vi "Action2Target.vi"() -> ()   [LabVIEW 2017]
panel:
  in  "Current":dbl
  in  "Target":dbl
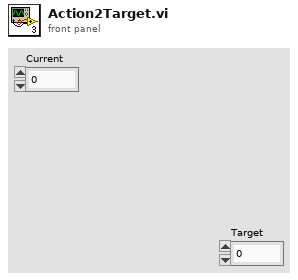
[diagram p1: front panel]
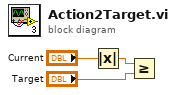
[diagram p0: block diagram]
diagram:
  n1 = Absolute Value(x="Current") -> (abs(x)=w2:dbl)
  n2 = Greater Or Equal?(x=w2, y="Target") -> ()  [unwired: 1 out]
